vi "take.vi"(2 "AWG index":u32, 3 "cluster":cluster{i32[][], i32[][], i32[][], i32[][]}) -> (0 "Array":i32[][](array[numeric]), 1 "output cluster":cluster{i32[][], i32[][], i32[][]})   [LabVIEW 2013]
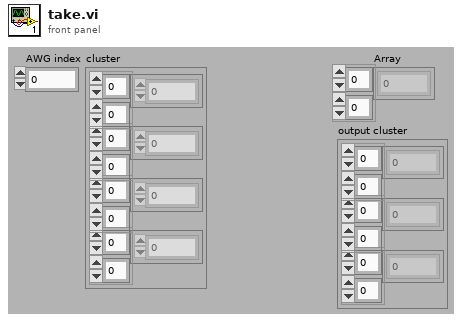
[diagram p1: front panel]
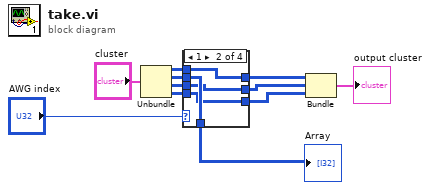
[diagram p0: block diagram]
diagram:
  n1 = Unbundle("cluster") -> (w11:i32[][], w10:i32[][], w9:i32[][], w8:i32[][])
  n2 = case shown="1" "AWG index" {
    tunnel: [w12 w17 w20 w25] -> w3
    tunnel: w11 -> [w15 w18 w23 w27]
    tunnel: w10 -> [w14 w19 w22 w26]
    tunnel: w9 -> [w13 w16 w21 w25]
    tunnel: w8 -> [w12 w17 w20 w24]
    tunnel: [w14 w18 w23 w27] -> w5
    tunnel: [w13 w16 w22 w26] -> w4
    tunnel: [w15 w19 w21 w24] -> w6
    frame 0, Default {
    }
    frame 1 {
    }
    frame 2 {
    }
    frame 3 {
    }
  }
  "Array" <- w6
  n3 = Bundle(w5, w4, w3) -> (→"output cluster":cluster{i32[][], i32[][], i32[][]})  [unwired: 1 in]
